vi "MS SQL_Open.vi"(6 "Bckup_DB?":bool, 8 "error in (no error)":errorcluster) -> (0 "error out":errorcluster, 3 "Ref Out":T1={"MS SQL Connection"=refnum, "UDL File"=path "", "Time"="", "DCODE"="", "WIP+1"=0, "MC No?"=0, "POKAYOKE?"=FALSE, "Expected Result"="", "Result [Status]"="", "Clock"=0.0, "RFID"="", "WIP Queue"=refnum, "TS Parameter"={"ProfitCenterCode"="", "LineCode"="", "WorkOrderNumber"="", "Model"="", "Model_with_Prefix"="", "VendorCode"="", "SetParameterDateCode"="", "PokaYoke"=0, "Target"=1, "Live_DateCode"="", "CustomerPartNumber"="", "Hand"="", "sBarcode"=FALSE, "FCA"=0, "Ent_Stamp"=timestamp(0 s since 1904-01-01), "STS_CD"=0.0}, "Data_Queue"=[], "RFID Serial No."=""} {"TS Parameter"."FCA" format="%01d"; "TS Parameter"."Target" min=1 max=100000; "TS Parameter"."PokaYoke" min=0 max=1}, 4 "element":string)   [LabVIEW 2020]
uses:
  Controls/TD SQL.ctl
  <vilib>/addons/database/Connection.llb/Conn ObjectReference.ctl
  Controls/WIP_State.ctl
  Controls/TS_Parameter.ctl
  <vilib>/addons/database/Connection.llb/DB Tools Open Connec (Path).vi
  <vilib>/addons/database/NI_Database_API.lvlib
panel:
  out "array":string[](array[string])
  out "ConnectionString":string
  out "path":path
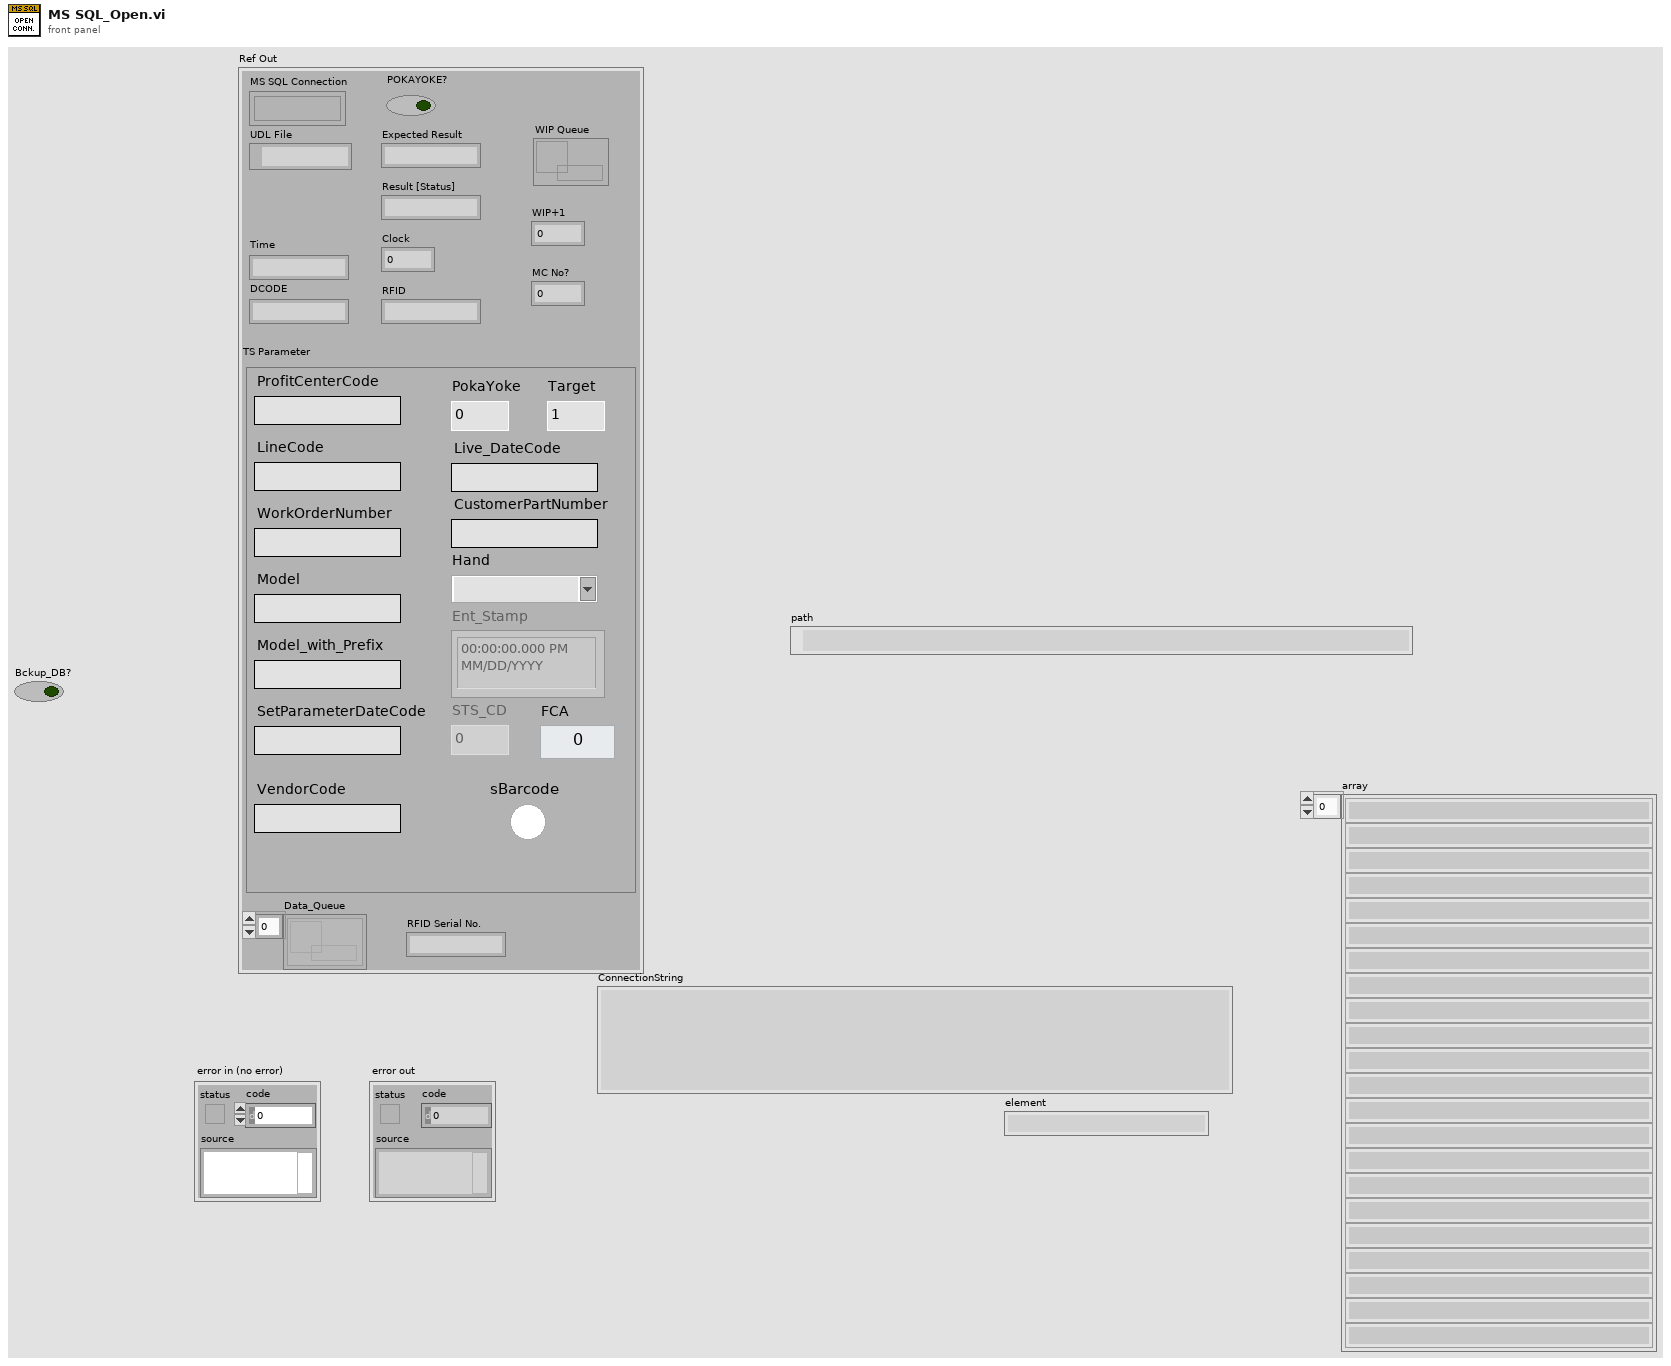
[diagram p1: front panel]
types:
  T1 = typedef "TD SQL.ctl" = cluster{"MS SQL Connection":T2, "UDL File":path, "Time":string, "DCODE":string, "WIP+1":i64, "MC No?":i32, "POKAYOKE?":bool, "Expected Result":string, "Result [Status]":string, "Clock":dbl, "RFID":string, "WIP Queue":refnum<queue>, "TS Parameter":T3, "Data_Queue":refnum<queue>[], "RFID Serial No.":string}
  T2 = typedef "NI_Database_API.lvlib/Conn ObjectReference.ctl" = refnum<k1>
  T3 = typedef "TS_Parameter.ctl" = cluster{"ProfitCenterCode":string, "LineCode":string, "WorkOrderNumber":string, "Model":string, "Model_with_Prefix":string, "VendorCode":string, "SetParameterDateCode":string, "PokaYoke":i32, "Target":i32, "Live_DateCode":string, "CustomerPartNumber":string, "Hand":string, "sBarcode":bool, "FCA":i32, "Ent_Stamp":timestamp, "STS_CD":dbl}
  T4 = typedef "NI_Database_API.lvlib/Conn DataMembers.ctl" = cluster{"ADODB._Connection":refnum<k7>, "recordset objects":i32, "command objects":i32}
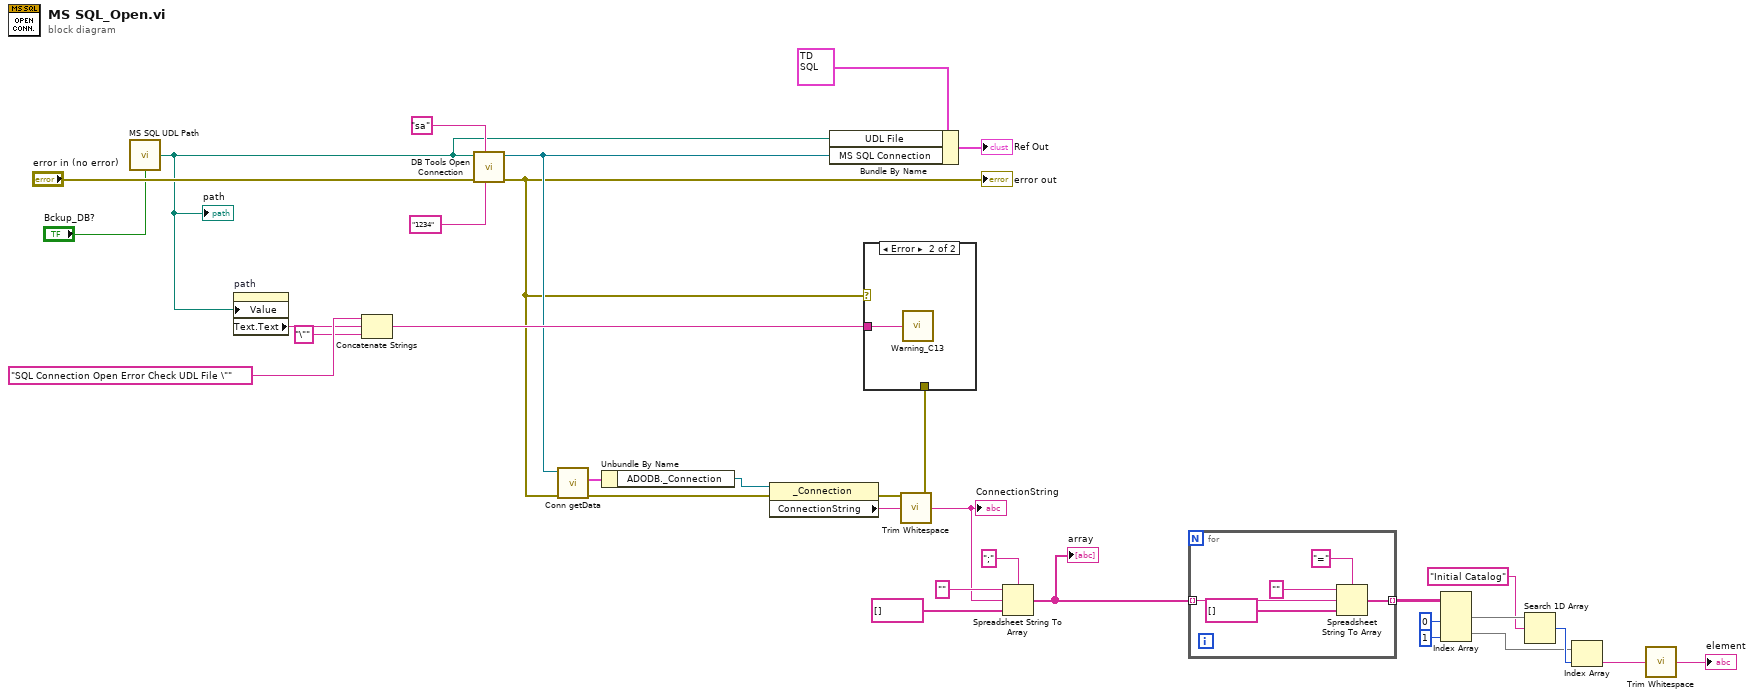
[diagram p0: block diagram]
diagram:
  n1 = call "MS SQL UDL Path.vi"("Bckup_DB?"="Bckup_DB?") -> ("UDL File Location"=w23:path)  [unwired: 3 in]
  "path" <- w23
  n2 = property on="path" class="Path"("Value"=w23) -> ("Text.Text"=w25:string)  [unwired: 2 in, 2 out]
  n3 = Concatenate Strings("SQL Connection Open Error Check UDL File \"" ("string"), w25, "\"" ("string")) -> (w26:string)
  n4 = call-poly <vilib>:"DB Tools Open Connection.vi"("password"="1234", "userID"="sa", "error in (no error)"="error in (no error)", "connection information"=w23) -> ("error out"=w17:errorcluster, "connection reference"=w20:T2)  [unwired: 4 in]
  "error out" <- w17
  n5 = call <vilib>:"Conn getData.vi"("error in (no error)"=w17, "connection reference"=w20) -> ("error out"=w18:errorcluster, "data"=w21:T4)  [unwired: 2 in, 2 out]
  n6 = Unbundle By Name(w21) -> ("ADODB._Connection"=w19:refnum<k7>)
  n7 = property class="_Connection"(reference=w19, error in=w18) -> (error out=w16:errorcluster, "ConnectionString"=w15:string)  [unwired: 1 out]
  n8 = Bundle By Name(cluster=T1 {"MS SQL Connection"=refnum, "UDL File"=path "", "Time"="", "DCODE"="", "WIP+1"=0, "MC No?"=0, "POKAYOKE?"=FALSE, "Expected Result"="", "Result [Status]"="", "Clock"=0.0, "RFID"="", "WIP Queue"=refnum, "TS Parameter"={"ProfitCenterCode"="", "LineCode"="", "WorkOrderNumber"="", "Model"="", "Model_with_Prefix"="", "VendorCode"="", "SetParameterDateCode"="", "PokaYoke"=0, "Target"=1, "Live_DateCode"="", "CustomerPartNumber"="", "Hand"="", "sBarcode"=FALSE, "FCA"=0, "Ent_Stamp"=timestamp(0 s since 1904-01-01), "STS_CD"=0.0}, "Data_Queue"=[], "RFID Serial No."=""} ("TD SQL"), "UDL File"=w23, "MS SQL Connection"=w20) -> (→"Ref Out":T1)
  n9 = case shown="Error" w17 {
    tunnel: w26 -> [_ w33]
    tunnel: w16 -> [_ _]
    frame No Error {
    }
    frame Error {
      n10 = call "Warning_C13.vi"("Warning in"=w33) -> ()  [unwired: 15 in]
    }
  }
  n11 = call <vilib>:"Trim Whitespace.vi"("string"=w15) -> ("trimmed string"=w11:string)  [unwired: 1 in]
  "ConnectionString" <- w11
  n12 = Spreadsheet String To Array(delimiter (Tab)=";", format string="" ("ConnectionString"), spreadsheet string=w11, array type (2D Dbl)=string[] []) -> (array=w10:string[])
  "array" <- w10
  n13 = for {
    tunnel: w10 -> [w35] mode=indexing
    tunnel: [w34] -> w9 mode=indexing
    n14 = Spreadsheet String To Array(delimiter (Tab)="=", format string="" ("ConnectionString"), spreadsheet string=w35, array type (2D Dbl)=string[] []) -> (array=w34:string[])
  }
  n15 = Index Array(array=w9, index (col) #1=0 ("disabled index (col)"), index (col) #2=1 ("index (col)")) -> (element #1=w6:string[], element #2=w3:string[])  [unwired: 2 in]
  n16 = Search 1D Array(1D array=w6, element="Initial Catalog" ("ConnectionString 2")) -> (index of element=w4:i32)  [unwired: 1 in]
  n17 = Index Array(array=w3, index=w4) -> (element=w2:string)
  n18 = call <vilib>:"Trim Whitespace.vi"("string"=w2) -> ("trimmed string"=→"element":string)  [unwired: 1 in]
